vi "Agilent 3458 Acquire And Chart Level Triggered.vi"() -> ()   [LabVIEW 2010]
doc: "Acquires and charts measurements caused by a level trigger. It does not implement math functions but can be added by the user."
uses:
  <instrlib>/Agilent 3458/Public/Data/Read Measurement(Multiple Points).vi
  <instrlib>/Agilent 3458/Agilent 3458.lvlib
panel:
  in  "Manual Range (1.00)":dbl=1.0 format="%_3g"
  in  "Maximum Time (10000 ms)":u32=10000
  in  "Trigger Count (1)":dbl=1.0
  in  "Enable Level Filtering (Enable)":bool=TRUE
  in  "Percentage (0%)":dbl
  in  "Slope (1:Positive)":u16(ring)=1 items=["Negative", "Positive"]
  in  "Coupling (0:AC)":u16(ring) items=["AC", "DC"]
  in  "Sample Count (1)":dbl=10.0 format="%#.6g"
  in  "Auto Range (1:ON)":u16(ring)=1 items=["OFF", "ON", "ONCE"]
  in  "Frequency Source (3: AC Voltage)":u16(ring)=3 items=["AC + DC Current", "AC + DC Voltage", "AC Current", "AC Voltage"]
  in  "Manual Resolution (2: 6.5 digits)":enum16{"4.5", "5.5", "6.5", "7.5", "8.5"}(ring)=enum."6.5"
  out "Waveform Chart":sgl[](graph)
  in  "VISA resource name":refnum<visa-resource-name>
  in  "Function (0: DC Voltage)":u16(ring) items=["DC Voltage", "AC Voltage", "AC + DC Voltage", "DC Current", "AC Current", "AC + DC Current", "2-Wire Resistance", "4-Wire Resistance", "Frequency", "Period", "Direct Sampling DC", "Direct Sampling AC"]
  # "(c) 2007  National Instruments.  ALL RIGHTS RESERVED."
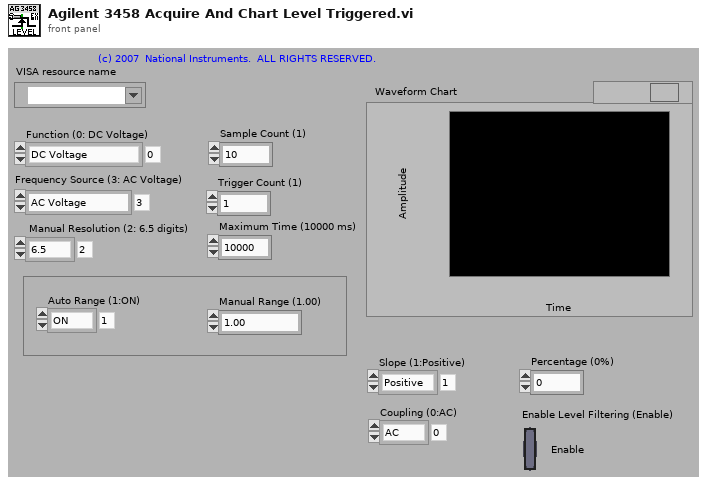
[diagram p1: front panel]
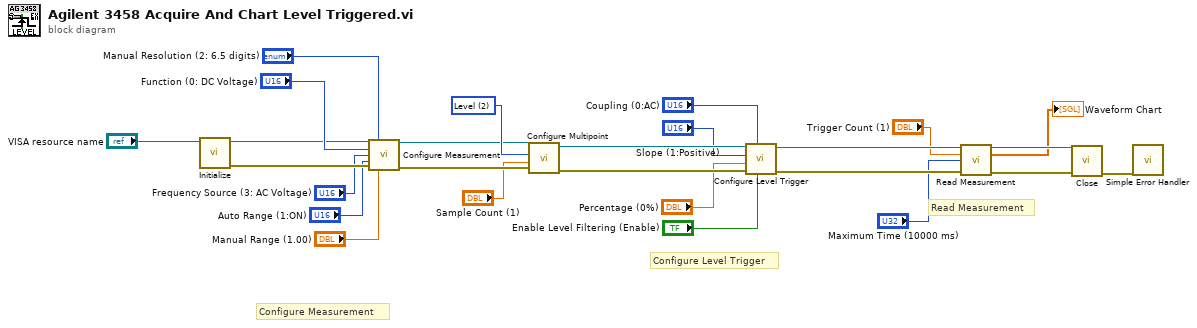
[diagram p0: block diagram]
diagram:
  w20 = u16 2 items=["Auto", "External", "Level", "Line", "Synchronous"] ("Trigger  Event(0:Auto)")
  # "Configure Level Trigger"
  # "Read Measurement"
  # "Configure Measurement"
  n1 = call <instrlib>:"Initialize.vi"("VISA resource name"="VISA resource name") -> ("error out"=w14:errorcluster, "VISA resource name out"=w15:refnum<visa-resource-name>)  [unwired: 9 in]
  n2 = call <instrlib>:"Configure Measurement.vi"("VISA resource name"=w15, "Manual Resolution (2: 6.5 digits)"="Manual Resolution (2: 6.5 digits)", "Function (0: DC Voltage)"="Function (0: DC Voltage)", "Frequency Source (3: AC Voltage)"="Frequency Source (3: AC Voltage)", "Auto Range (1:ON)"="Auto Range (1:ON)", "error in (no error)"=w14, "Manual Range (1.00)"="Manual Range (1.00)") -> ("VISA resource name out"=w19:refnum<visa-resource-name>, "error out"=w18:errorcluster)  [unwired: 7 in]
  n3 = call <instrlib>:"Configure Multipoint.vi"("error in (no error)"=w18, "Sample Count (1)"="Sample Count (1)", "Trigger Type (0:Auto)"=w20, "VISA resource name"=w19) -> ("error out"=w16:errorcluster, "VISA resource name out"=w17:refnum<visa-resource-name>)  [unwired: 6 in]
  n4 = call <instrlib>:"Configure Level Trigger.vi"("Enable Level Filtering (Enable)"="Enable Level Filtering (Enable)", "Coupling (0:AC)"="Coupling (0:AC)", "error in (no error)"=w16, "Percentage (0%)"="Percentage (0%)", "Slope (1:Positive)"="Slope (1:Positive)", "VISA resource name"=w17) -> ("error out"=w11:errorcluster, "VISA resource name out"=w12:refnum<visa-resource-name>)  [unwired: 4 in]
  n5 = call-poly <instrlib>:"Read Measurement.vi"("VISA resource name"=w12, "Trigger Count (1)"="Trigger Count (1)", "Maximum Time (10000 ms)"="Maximum Time (10000 ms)", "error in (no error)"=w11) -> ("VISA resource name out"=w26:refnum<visa-resource-name>, "Measurements"=→"Waveform Chart":sgl[], "error out"=w25:errorcluster)  [unwired: 9 in]
  n6 = call <instrlib>:"Close.vi"("error in (no error)"=w25, "VISA resource name"=w26) -> ("error out"=w24:errorcluster)  [unwired: 9 in]
  n7 = call <vilib>:"Simple Error Handler.vi"("error in (no error)"=w24) -> ()  [unwired: 4 in, 5 out]
